vi "Insert Into Array (Multi String).vi"(9 "index":i32, 10 "Array":string[](array[string]), 11 "JSON Array in":refnum<class "JSON Helper.lvclass">) -> (3 "JSON Array out":refnum<class "JSON Helper.lvclass">)   [LabVIEW 2016, in "JSON Helper.lvclass"]
doc: "Inserts an element or subarray into a JSON array at the point you specify in index."
uses:
  JSON Helper/JSON Helper.lvclass
  JSON String/New JSON String.vi
  Insert Into Array (Multi).vi
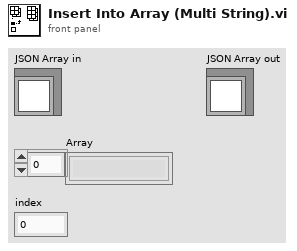
[diagram p1: front panel]
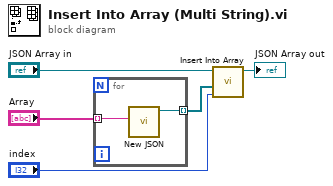
[diagram p0: block diagram]
diagram:
  n1 = for {
    tunnel: "Array" -> [w7] mode=indexing
    tunnel: [w6] -> w2 mode=indexing
    n2 = call-poly "New JSON.vi"("value"=w7) -> ("JSON String out"=w6:refnum<class "JSON Helper.lvclass">)  [unwired: 9 in, 1 out]
  }
  n3 = call-poly "Insert Into Array.vi"("index"="index", "Array"=w2, "JSON Array in"="JSON Array in") -> ("JSON Array out"=→"JSON Array out":refnum<class "JSON Helper.lvclass">)  [unwired: 8 in]
